vi "Activity_12.vi"() -> ()   [LabVIEW 2015]
panel:
  in  "stop":bool
  out "Boolean 5":bool
  out "Boolean 4":bool
  out "Boolean 3":bool
  out "Boolean 2":bool
  out "Boolean":bool
  out "Terminal1":string
  out "Terminal2":string
  out "Terminal3":string
  out "Terminal4":string
  out "Terminal5":string
  out "Destino2":string
  out "Destino5":string
  out "Destino4":string
  out "Destino3":string
  out "Destino1":string
  out "Aerolinea5":u16(ring)
  out "Aerolinea4":u16(ring)
  out "Aerolinea3":u16(ring)
  out "Aerolinea2":u16(ring)
  out "Aerolinea":u16(ring)
  out "String 2":string
  out "String":string
  # "Simulador de Tablero de Anuncios de Vuelo"
  # "Serrano Bermúdez Luis Esteban\nFecha de Entrega 02/03/2019"
  # "Descripción:"
  # "Simula la llegada y salida de vuelos en un Aeropuerto, muestra\nel destino, la aerolinea, el estatus del vuelo y la terminal del vuelo\nHace un restraso de 5 seg. entre cada cambio de estado"
  # "Destino"
  # "Terminal"
  # "Aerolinea"
  # "Estatus"
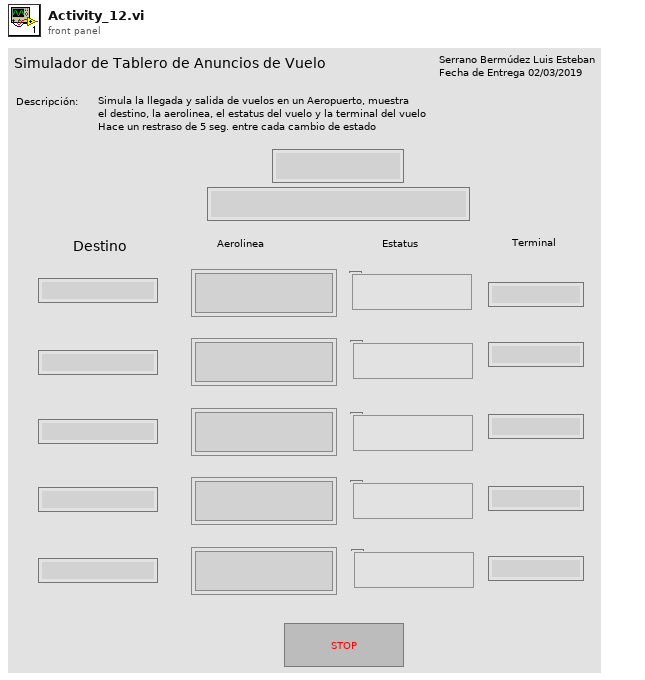
[diagram p1: front panel]
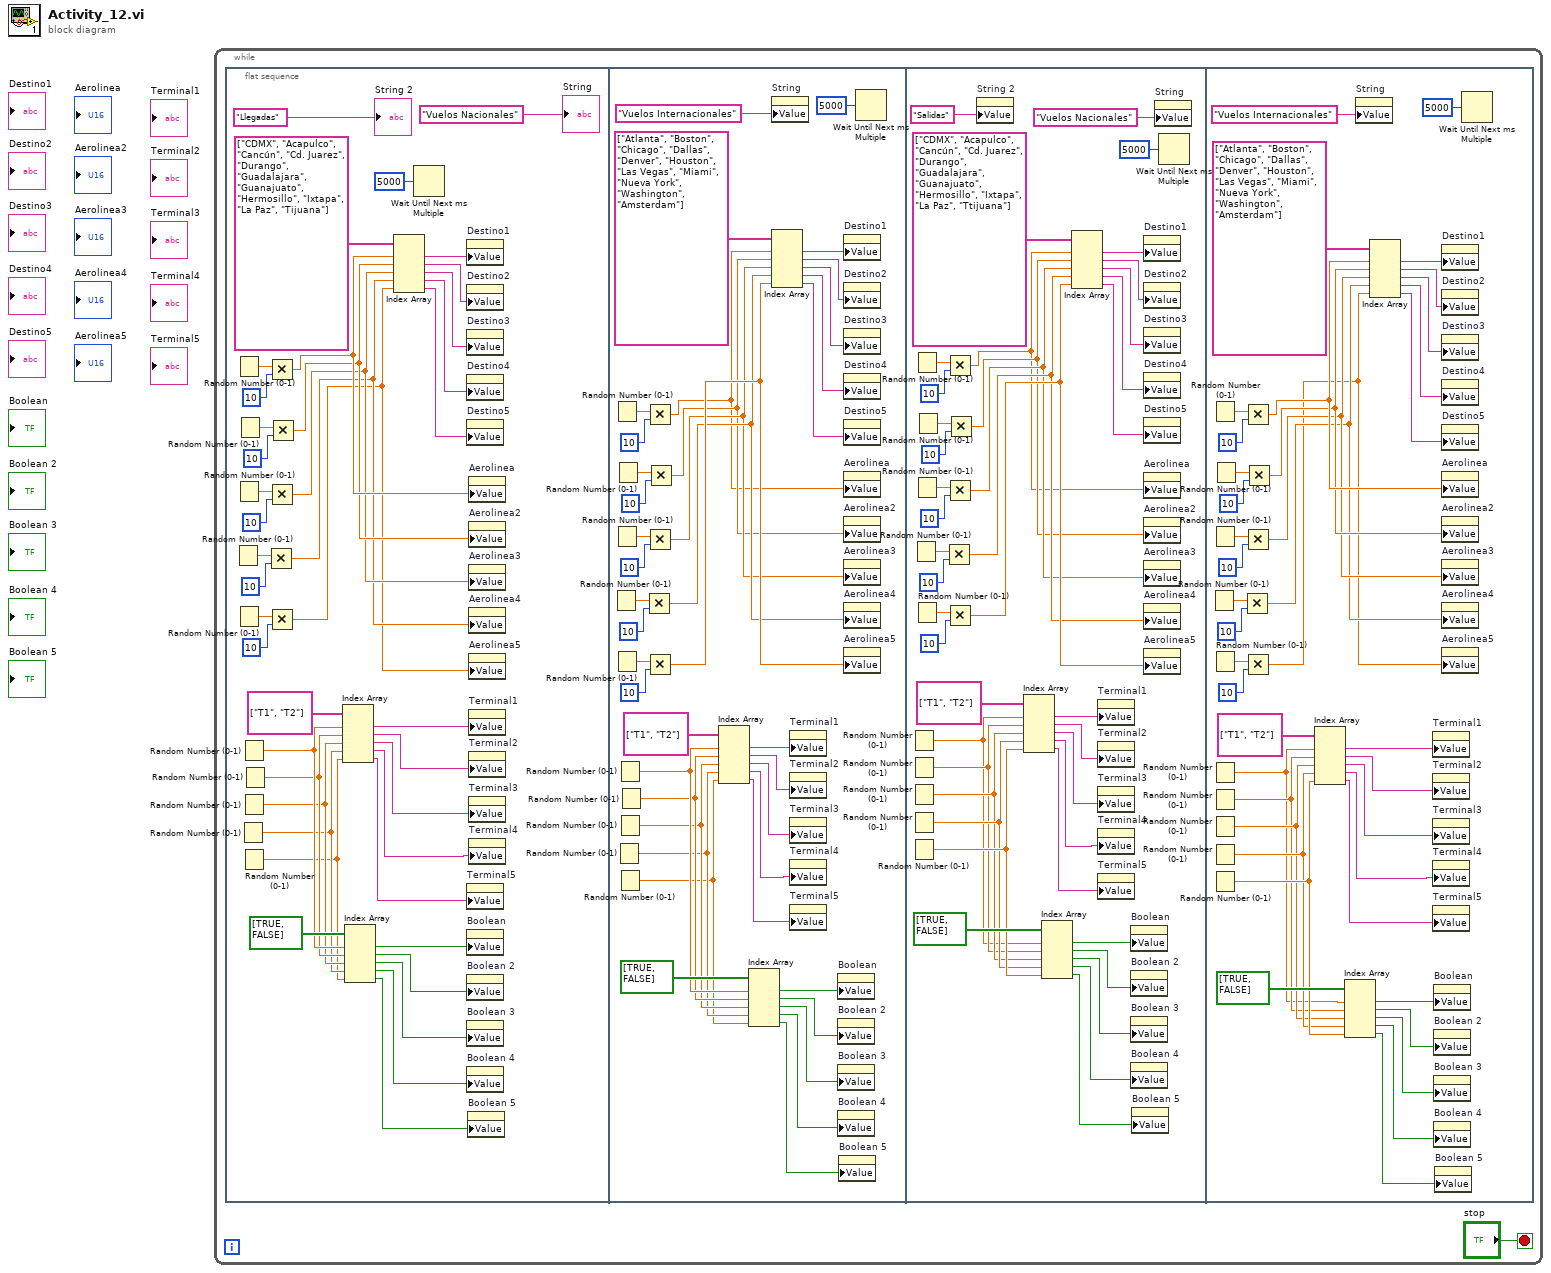
[diagram p0: block diagram]
diagram:
  n1 = while {
    stop <- "stop" stop-if-true
    n2 = flat-sequence {
      frame #0 {
        n3 = Random Number (0-1)() -> (number: 0 to 1=w34:dbl)
        n4 = Random Number (0-1)() -> (number: 0 to 1=w26:dbl)
        n5 = Random Number (0-1)() -> (number: 0 to 1=w30:dbl)
        n6 = Random Number (0-1)() -> (number: 0 to 1=w32:dbl)
        n7 = Random Number (0-1)() -> (number: 0 to 1=w29:dbl)
        n8 = Random Number (0-1)() -> (number: 0 to 1=w8:dbl)
        n9 = Random Number (0-1)() -> (number: 0 to 1=w11:dbl)
        n10 = Random Number (0-1)() -> (number: 0 to 1=w9:dbl)
        n11 = Random Number (0-1)() -> (number: 0 to 1=w7:dbl)
        n12 = Random Number (0-1)() -> (number: 0 to 1=w10:dbl)
        n13 = Multiply(x=w34, y=10) -> (x*y=w20:dbl)
        n14 = Multiply(x=w26, y=10) -> (x*y=w23:dbl)
        n15 = Multiply(x=w30, y=10) -> (x*y=w21:dbl)
        n16 = Multiply(x=w32, y=10) -> (x*y=w19:dbl)
        n17 = Multiply(x=w29, y=10) -> (x*y=w22:dbl)
        n18 = Index Array(array=string[] ["T1", "T2"], index #1=w11, index #2=w10, index #3=w9, index #4=w8, index #5=w7) -> (element #1=w17:string, element #2=w16:string, element #3=w13:string, element #4=w14:string, element #5=w15:string)
        n19 = Index Array(array=bool[] [TRUE, FALSE], index #1=w11, index #2=w10, index #3=w9, index #4=w8, index #5=w7) -> (element #1=w6:bool, element #2=w5:bool, element #3=w2:bool, element #4=w3:bool, element #5=w4:bool)
        n20 = Index Array(array=string[] ["CDMX", "Acapulco", "Cancún", "Cd. Juarez", "Durango", "Guadalajara", "Guanajuato", "Hermosillo", "Ixtapa", "La Paz", "Tijuana"], index #1=w23, index #2=w22, index #3=w21, index #4=w20, index #5=w19) -> (element #1=w35:string, element #2=w36:string, element #3=w37:string, element #4=w38:string, element #5=w39:string)
        n21 = Wait Until Next ms Multiple(millisecond multiple=u32 5000) -> ()  [unwired: 1 out]
        n22 = property on="Destino1" class="Str"("Value"=w35) -> ()  [unwired: 2 in, 2 out]
        n23 = property on="Destino2" class="Str"("Value"=w36) -> ()  [unwired: 2 in, 2 out]
        n24 = property on="Destino3" class="Str"("Value"=w37) -> ()  [unwired: 2 in, 2 out]
        n25 = property on="Destino4" class="Str"("Value"=w38) -> ()  [unwired: 2 in, 2 out]
        n26 = property on="Destino5" class="Str"("Value"=w39) -> ()  [unwired: 2 in, 2 out]
        n27 = property on="Terminal5" class="Str"("Value"=w15) -> ()  [unwired: 2 in, 2 out]
        n28 = property on="Boolean" class="Bool (strict)"("Value"=w6) -> ()  [unwired: 2 in, 2 out]
        n29 = property on="Boolean 2" class="Bool (strict)"("Value"=w5) -> ()  [unwired: 2 in, 2 out]
        n30 = property on="Boolean 3" class="Bool (strict)"("Value"=w2) -> ()  [unwired: 2 in, 2 out]
        n31 = property on="Boolean 4" class="Bool (strict)"("Value"=w3) -> ()  [unwired: 2 in, 2 out]
        n32 = property on="Boolean 5" class="Bool (strict)"("Value"=w4) -> ()  [unwired: 2 in, 2 out]
        n33 = property on="Aerolinea" class="Ring (strict)"("Value"=w23) -> ()  [unwired: 2 in, 2 out]
        n34 = property on="Aerolinea2" class="Ring (strict)"("Value"=w22) -> ()  [unwired: 2 in, 2 out]
        n35 = property on="Aerolinea3" class="Ring (strict)"("Value"=w21) -> ()  [unwired: 2 in, 2 out]
        n36 = property on="Aerolinea4" class="Ring (strict)"("Value"=w20) -> ()  [unwired: 2 in, 2 out]
        n37 = property on="Aerolinea5" class="Ring (strict)"("Value"=w19) -> ()  [unwired: 2 in, 2 out]
        n38 = property on="Terminal1" class="Str"("Value"=w17) -> ()  [unwired: 2 in, 2 out]
        n39 = property on="Terminal2" class="Str"("Value"=w16) -> ()  [unwired: 2 in, 2 out]
        n40 = property on="Terminal3" class="Str"("Value"=w13) -> ()  [unwired: 2 in, 2 out]
        n41 = property on="Terminal4" class="Str"("Value"=w14) -> ()  [unwired: 2 in, 2 out]
        "String" <- "Vuelos Nacionales"
        "String 2" <- "Llegadas"
      }
      frame #1 {
        n42 = Random Number (0-1)() -> (number: 0 to 1=w67:dbl)
        n43 = Random Number (0-1)() -> (number: 0 to 1=w75:dbl)
        n44 = Random Number (0-1)() -> (number: 0 to 1=w71:dbl)
        n45 = Random Number (0-1)() -> (number: 0 to 1=w69:dbl)
        n46 = Random Number (0-1)() -> (number: 0 to 1=w72:dbl)
        n47 = Random Number (0-1)() -> (number: 0 to 1=w44:dbl)
        n48 = Random Number (0-1)() -> (number: 0 to 1=w47:dbl)
        n49 = Random Number (0-1)() -> (number: 0 to 1=w45:dbl)
        n50 = Random Number (0-1)() -> (number: 0 to 1=w43:dbl)
        n51 = Random Number (0-1)() -> (number: 0 to 1=w46:dbl)
        n52 = Multiply(x=w67, y=10) -> (x*y=w80:dbl)
        n53 = Multiply(x=w75, y=10) -> (x*y=w77:dbl)
        n54 = Multiply(x=w71, y=10) -> (x*y=w79:dbl)
        n55 = Multiply(x=w69, y=10) -> (x*y=w81:dbl)
        n56 = Multiply(x=w72, y=10) -> (x*y=w78:dbl)
        n57 = Index Array(array=string[] ["T1", "T2"], index #1=w47, index #2=w46, index #3=w45, index #4=w44, index #5=w43) -> (element #1=w55:string, element #2=w56:string, element #3=w59:string, element #4=w58:string, element #5=w57:string)
        n58 = Index Array(array=bool[] [TRUE, FALSE], index #1=w47, index #2=w46, index #3=w45, index #4=w44, index #5=w43) -> (element #1=w49:bool, element #2=w50:bool, element #3=w53:bool, element #4=w52:bool, element #5=w51:bool)
        n59 = property on="String" class="Str"("Value"="Vuelos Internacionales") -> ()  [unwired: 2 in, 2 out]
        n60 = Index Array(array=string[] ["Atlanta", "Boston", "Chicago", "Dallas", "Denver", "Houston", "Las Vegas", "Miami", "Nueva York", "Washington", "Amsterdam"], index #1=w77, index #2=w78, index #3=w79, index #4=w80, index #5=w81) -> (element #1=w66:string, element #2=w65:string, element #3=w64:string, element #4=w63:string, element #5=w62:string)
        n61 = property on="Terminal1" class="Str"("Value"=w55) -> ()  [unwired: 2 in, 2 out]
        n62 = property on="Terminal2" class="Str"("Value"=w56) -> ()  [unwired: 2 in, 2 out]
        n63 = property on="Terminal3" class="Str"("Value"=w59) -> ()  [unwired: 2 in, 2 out]
        n64 = property on="Terminal4" class="Str"("Value"=w58) -> ()  [unwired: 2 in, 2 out]
        n65 = property on="Terminal5" class="Str"("Value"=w57) -> ()  [unwired: 2 in, 2 out]
        n66 = property on="Boolean" class="Bool (strict)"("Value"=w49) -> ()  [unwired: 2 in, 2 out]
        n67 = property on="Boolean 2" class="Bool (strict)"("Value"=w50) -> ()  [unwired: 2 in, 2 out]
        n68 = property on="Boolean 3" class="Bool (strict)"("Value"=w53) -> ()  [unwired: 2 in, 2 out]
        n69 = property on="Boolean 4" class="Bool (strict)"("Value"=w52) -> ()  [unwired: 2 in, 2 out]
        n70 = property on="Boolean 5" class="Bool (strict)"("Value"=w51) -> ()  [unwired: 2 in, 2 out]
        n71 = property on="Destino1" class="Str"("Value"=w66) -> ()  [unwired: 2 in, 2 out]
        n72 = property on="Destino2" class="Str"("Value"=w65) -> ()  [unwired: 2 in, 2 out]
        n73 = property on="Destino3" class="Str"("Value"=w64) -> ()  [unwired: 2 in, 2 out]
        n74 = property on="Destino4" class="Str"("Value"=w63) -> ()  [unwired: 2 in, 2 out]
        n75 = property on="Destino5" class="Str"("Value"=w62) -> ()  [unwired: 2 in, 2 out]
        n76 = property on="Aerolinea" class="Ring (strict)"("Value"=w77) -> ()  [unwired: 2 in, 2 out]
        n77 = property on="Aerolinea2" class="Ring (strict)"("Value"=w78) -> ()  [unwired: 2 in, 2 out]
        n78 = property on="Aerolinea3" class="Ring (strict)"("Value"=w79) -> ()  [unwired: 2 in, 2 out]
        n79 = property on="Aerolinea4" class="Ring (strict)"("Value"=w80) -> ()  [unwired: 2 in, 2 out]
        n80 = property on="Aerolinea5" class="Ring (strict)"("Value"=w81) -> ()  [unwired: 2 in, 2 out]
        n81 = Wait Until Next ms Multiple(millisecond multiple=u32 5000) -> ()  [unwired: 1 out]
      }
      frame #2 {
        n82 = Random Number (0-1)() -> (number: 0 to 1=w83:dbl)
        n83 = Random Number (0-1)() -> (number: 0 to 1=w84:dbl)
        n84 = Random Number (0-1)() -> (number: 0 to 1=w85:dbl)
        n85 = Random Number (0-1)() -> (number: 0 to 1=w86:dbl)
        n86 = Random Number (0-1)() -> (number: 0 to 1=w87:dbl)
        n87 = Random Number (0-1)() -> (number: 0 to 1=w106:dbl)
        n88 = Random Number (0-1)() -> (number: 0 to 1=w114:dbl)
        n89 = Random Number (0-1)() -> (number: 0 to 1=w110:dbl)
        n90 = Random Number (0-1)() -> (number: 0 to 1=w108:dbl)
        n91 = Random Number (0-1)() -> (number: 0 to 1=w111:dbl)
        n92 = Multiply(x=w106, y=10) -> (x*y=w120:dbl)
        n93 = Multiply(x=w114, y=10) -> (x*y=w117:dbl)
        n94 = Multiply(x=w110, y=10) -> (x*y=w119:dbl)
        n95 = Multiply(x=w108, y=10) -> (x*y=w121:dbl)
        n96 = Multiply(x=w111, y=10) -> (x*y=w118:dbl)
        n97 = property on="String 2" class="Str"("Value"="Salidas") -> ()  [unwired: 2 in, 2 out]
        n98 = Index Array(array=string[] ["T1", "T2"], index #1=w83, index #2=w84, index #3=w85, index #4=w86, index #5=w87) -> (element #1=w98:string, element #2=w97:string, element #3=w94:string, element #4=w95:string, element #5=w96:string)
        n99 = Index Array(array=bool[] [TRUE, FALSE], index #1=w83, index #2=w84, index #3=w85, index #4=w86, index #5=w87) -> (element #1=w92:bool, element #2=w91:bool, element #3=w88:bool, element #4=w89:bool, element #5=w90:bool)
        n100 = Index Array(array=string[] ["CDMX", "Acapulco", "Cancún", "Cd. Juarez", "Durango", "Guadalajara", "Guanajuato", "Hermosillo", "Ixtapa", "La Paz", "Ttijuana"], index #1=w117, index #2=w118, index #3=w119, index #4=w120, index #5=w121) -> (element #1=w105:string, element #2=w104:string, element #3=w103:string, element #4=w102:string, element #5=w101:string)
        n101 = property on="Terminal1" class="Str"("Value"=w98) -> ()  [unwired: 2 in, 2 out]
        n102 = property on="Terminal2" class="Str"("Value"=w97) -> ()  [unwired: 2 in, 2 out]
        n103 = property on="Terminal3" class="Str"("Value"=w94) -> ()  [unwired: 2 in, 2 out]
        n104 = property on="Terminal4" class="Str"("Value"=w95) -> ()  [unwired: 2 in, 2 out]
        n105 = property on="Terminal5" class="Str"("Value"=w96) -> ()  [unwired: 2 in, 2 out]
        n106 = property on="Boolean" class="Bool (strict)"("Value"=w92) -> ()  [unwired: 2 in, 2 out]
        n107 = property on="Boolean 2" class="Bool (strict)"("Value"=w91) -> ()  [unwired: 2 in, 2 out]
        n108 = property on="Boolean 3" class="Bool (strict)"("Value"=w88) -> ()  [unwired: 2 in, 2 out]
        n109 = property on="Boolean 4" class="Bool (strict)"("Value"=w89) -> ()  [unwired: 2 in, 2 out]
        n110 = property on="Boolean 5" class="Bool (strict)"("Value"=w90) -> ()  [unwired: 2 in, 2 out]
        n111 = property on="Destino1" class="Str"("Value"=w105) -> ()  [unwired: 2 in, 2 out]
        n112 = property on="Destino2" class="Str"("Value"=w104) -> ()  [unwired: 2 in, 2 out]
        n113 = property on="Destino3" class="Str"("Value"=w103) -> ()  [unwired: 2 in, 2 out]
        n114 = property on="Destino4" class="Str"("Value"=w102) -> ()  [unwired: 2 in, 2 out]
        n115 = property on="Destino5" class="Str"("Value"=w101) -> ()  [unwired: 2 in, 2 out]
        n116 = property on="Aerolinea" class="Ring (strict)"("Value"=w117) -> ()  [unwired: 2 in, 2 out]
        n117 = property on="Aerolinea2" class="Ring (strict)"("Value"=w118) -> ()  [unwired: 2 in, 2 out]
        n118 = property on="Aerolinea3" class="Ring (strict)"("Value"=w119) -> ()  [unwired: 2 in, 2 out]
        n119 = property on="Aerolinea4" class="Ring (strict)"("Value"=w120) -> ()  [unwired: 2 in, 2 out]
        n120 = property on="Aerolinea5" class="Ring (strict)"("Value"=w121) -> ()  [unwired: 2 in, 2 out]
        n121 = property on="String" class="Str"("Value"="Vuelos Nacionales") -> ()  [unwired: 2 in, 2 out]
        n122 = Wait Until Next ms Multiple(millisecond multiple=u32 5000) -> ()  [unwired: 1 out]
      }
      frame #3 {
        n123 = Random Number (0-1)() -> (number: 0 to 1=w156:dbl)
        n124 = Random Number (0-1)() -> (number: 0 to 1=w148:dbl)
        n125 = Random Number (0-1)() -> (number: 0 to 1=w152:dbl)
        n126 = Random Number (0-1)() -> (number: 0 to 1=w154:dbl)
        n127 = Random Number (0-1)() -> (number: 0 to 1=w124:dbl)
        n128 = Random Number (0-1)() -> (number: 0 to 1=w125:dbl)
        n129 = Random Number (0-1)() -> (number: 0 to 1=w126:dbl)
        n130 = Random Number (0-1)() -> (number: 0 to 1=w127:dbl)
        n131 = Random Number (0-1)() -> (number: 0 to 1=w128:dbl)
        n132 = Random Number (0-1)() -> (number: 0 to 1=w151:dbl)
        n133 = Multiply(x=w156, y=10) -> (x*y=w143:dbl)
        n134 = Multiply(x=w148, y=10) -> (x*y=w146:dbl)
        n135 = Multiply(x=w152, y=10) -> (x*y=w144:dbl)
        n136 = Multiply(x=w154, y=10) -> (x*y=w142:dbl)
        n137 = Multiply(x=w151, y=10) -> (x*y=w145:dbl)
        n138 = Index Array(array=string[] ["T1", "T2"], index #1=w124, index #2=w125, index #3=w126, index #4=w127, index #5=w128) -> (element #1=w136:string, element #2=w137:string, element #3=w140:string, element #4=w139:string, element #5=w138:string)
        n139 = Index Array(array=bool[] [TRUE, FALSE], index #1=w124, index #2=w125, index #3=w126, index #4=w127, index #5=w128) -> (element #1=w130:bool, element #2=w131:bool, element #3=w134:bool, element #4=w133:bool, element #5=w132:bool)
        n140 = property on="String" class="Str"("Value"="Vuelos Internacionales") -> ()  [unwired: 2 in, 2 out]
        n141 = Index Array(array=string[] ["Atlanta", "Boston", "Chicago", "Dallas", "Denver", "Houston", "Las Vegas", "Miami", "Nueva York", "Washington", "Amsterdam"], index #1=w146, index #2=w145, index #3=w144, index #4=w143, index #5=w142) -> (element #1=w157:string, element #2=w158:string, element #3=w159:string, element #4=w160:string, element #5=w161:string)
        n142 = property on="Terminal1" class="Str"("Value"=w136) -> ()  [unwired: 2 in, 2 out]
        n143 = property on="Terminal2" class="Str"("Value"=w137) -> ()  [unwired: 2 in, 2 out]
        n144 = property on="Terminal3" class="Str"("Value"=w140) -> ()  [unwired: 2 in, 2 out]
        n145 = property on="Terminal4" class="Str"("Value"=w139) -> ()  [unwired: 2 in, 2 out]
        n146 = property on="Terminal5" class="Str"("Value"=w138) -> ()  [unwired: 2 in, 2 out]
        n147 = property on="Boolean" class="Bool (strict)"("Value"=w130) -> ()  [unwired: 2 in, 2 out]
        n148 = property on="Boolean 2" class="Bool (strict)"("Value"=w131) -> ()  [unwired: 2 in, 2 out]
        n149 = property on="Boolean 3" class="Bool (strict)"("Value"=w134) -> ()  [unwired: 2 in, 2 out]
        n150 = property on="Boolean 4" class="Bool (strict)"("Value"=w133) -> ()  [unwired: 2 in, 2 out]
        n151 = property on="Boolean 5" class="Bool (strict)"("Value"=w132) -> ()  [unwired: 2 in, 2 out]
        n152 = property on="Destino1" class="Str"("Value"=w157) -> ()  [unwired: 2 in, 2 out]
        n153 = property on="Destino2" class="Str"("Value"=w158) -> ()  [unwired: 2 in, 2 out]
        n154 = property on="Destino3" class="Str"("Value"=w159) -> ()  [unwired: 2 in, 2 out]
        n155 = property on="Destino4" class="Str"("Value"=w160) -> ()  [unwired: 2 in, 2 out]
        n156 = property on="Destino5" class="Str"("Value"=w161) -> ()  [unwired: 2 in, 2 out]
        n157 = property on="Aerolinea" class="Ring (strict)"("Value"=w146) -> ()  [unwired: 2 in, 2 out]
        n158 = property on="Aerolinea2" class="Ring (strict)"("Value"=w145) -> ()  [unwired: 2 in, 2 out]
        n159 = property on="Aerolinea3" class="Ring (strict)"("Value"=w144) -> ()  [unwired: 2 in, 2 out]
        n160 = property on="Aerolinea4" class="Ring (strict)"("Value"=w143) -> ()  [unwired: 2 in, 2 out]
        n161 = property on="Aerolinea5" class="Ring (strict)"("Value"=w142) -> ()  [unwired: 2 in, 2 out]
        n162 = Wait Until Next ms Multiple(millisecond multiple=u32 5000) -> ()  [unwired: 1 out]
      }
    }
  }
